vi "TestClientStreaming.vi"() -> ()   [LabVIEW 2019]
uses:
  Servers/TestDataMarshal/TestDataMarshal Class/RPC Messages/queryserver_ServerEvent/queryserver_ServerEvent_Data.ctl
  Servers/TestDataMarshal/TestDataMarshal Class/RPC Messages/queryserver_QueryRequest/queryserver_QueryRequest_Data.ctl
  3ce8af61-1d11-4712-b0ef-57def0cc284f.vi
  8ef641a7-92dd-4bb4-a86c-ef6a01ef9b17.vi
  labview source/gRPC lv Support/Server API/Server/Get Server DLL Path.vi
  labview source/gRPC lv Support/gprc-lvsupport.lvlib
  Servers/TestDataMarshal/TestDataMarshal Class/TestDataMarshal.lvclass
panel:
  out "Response Data":T1
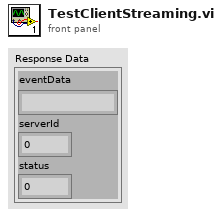
[diagram p1: front panel]
types:
  T1 = typedef "TestDataMarshal.lvlib/TestDataMarshal.lvclass/queryserver_ServerEvent_Data.ctl" = cluster{"eventData":string, "serverId":i32, "status":i32}
  T2 = typedef "TestDataMarshal.lvlib/TestDataMarshal.lvclass/queryserver_QueryRequest_Data.ctl" = cluster{"query":string}
  T3 = typedef "gprc-lvsupport.lvlib/grpcId.ctl" = u64
  T4 = typedef "TestDataMarshal.lvlib/gprc-lvsupport.lvlib/grpcId.ctl" = u64
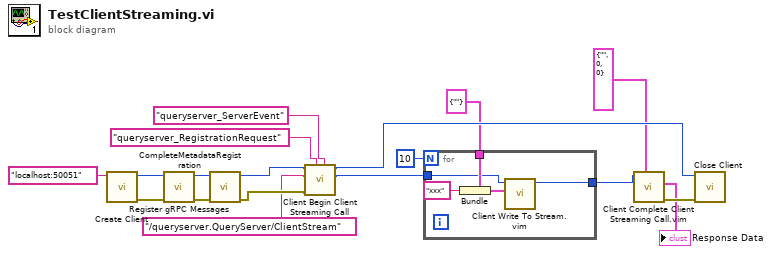
[diagram p0: block diagram]
diagram:
  n1 = call "Create Client.vi"("address"="localhost:50051") -> ("error out"=w15:errorcluster, "Client Ref Out"=w18:T3)  [unwired: 9 in]
  n2 = call "Register gRPC Messages.vi"("error in (no error)"=w15, "gRPC ID"=w18) -> ("error out"=w14:errorcluster, "gRPC ID Out"=w17:T4)  [unwired: 8 in]
  n3 = call "CompleteMetadataRegistration.vi"("error in (no error)"=w14, "gRPC ID"=w17) -> ("error out"=w12:errorcluster, "gRPC ID Out"=w8:T3)  [unwired: 8 in]
  n4 = call "Client Begin Client Streaming Call.vi"("Response Message Name"="queryserver_ServerEvent", "Request Message Name"="queryserver_RegistrationRequest", "error in (no error)"=w12, "Method Name"="/queryserver.QueryServer/ClientStream", "Client Ref"=w8) -> ("Call Id Out"=w6:T3, "Client Ref Out"=w13:T3)  [unwired: 4 in, 1 out]
  n5 = for {
    N: 10 -> [_]
    tunnel: T2 {"query"=""} ("queryserver_QueryRequest_Data") -> [w23]
    tunnel: w6 -> [w20]
    tunnel: [w19] -> w5
    n6 = Bundle(cluster=w23, "query"="xxx" ("eventData")) -> (w21:T2)
    n7 = call "Client Write To Stream.vim"("Request Data"=w21, "Call Id In"=w20) -> ("Call Id Out"=w19:u64)  [unwired: 7 in, 2 out]
  }
  n8 = call "Client Complete Client Streaming Call.vim"("Response Type"=T1 {"eventData"="", "serverId"=0, "status"=0} ("queryserver_ServerEvent_Data"), "Call Id"=w5) -> ("error out"=w4:errorcluster, "Response Data"=→"Response Data":T1)  [unwired: 7 in, 1 out]
  n9 = call "Close Client.vi"("error in (no error)"=w4, "Client Ref"=w13) -> ()  [unwired: 9 in, 1 out]
